vi "UTILITY Build Save Array.vi"(8 "Error In":errorcluster, 10 "New Header Save Array":T1[](array[typedef]), 11 "Full Data Array Out":string[][](array[string])) -> (0 "Error Out":errorcluster, 3 "Selected Data Array Out":string[][](array[string]))   [LabVIEW 2016]
uses:
  Washer DOE/Type Definitions/DOE Data Save Modifier.ctl
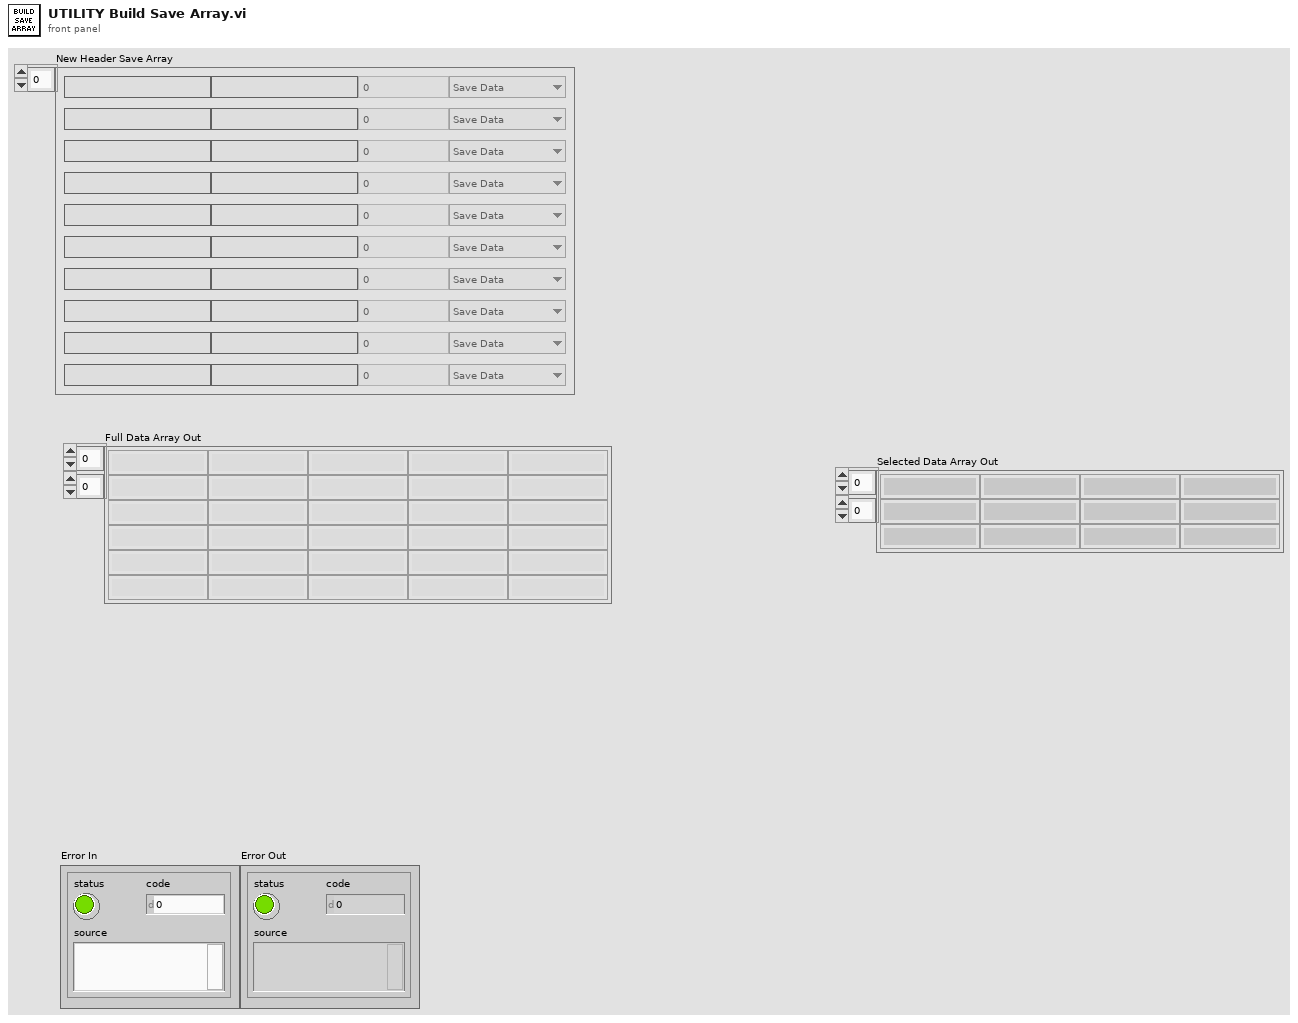
[diagram p1: front panel]
types:
  T1 = typedef "DOE Data Save Modifier.ctl" = cluster{"Name":string, "Title":string, "Save Status":enum16{"Save Data", "Don't Save Data"}, "Group":u8, "Field":u8}
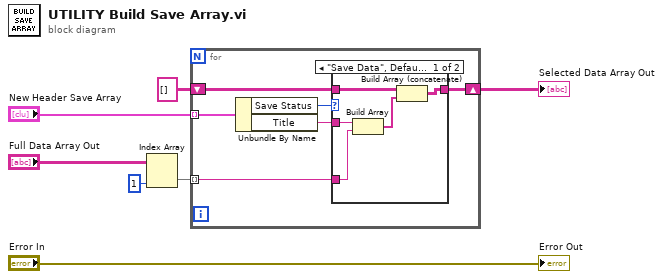
[diagram p0: block diagram]
diagram:
  n1 = Index Array(array="Full Data Array Out", index (col)=1 ("index (row)")) -> (element=w3:string[])  [unwired: 1 in]
  n2 = for {
    tunnel: "New Header Save Array" -> [w13] mode=indexing
    shift-right: [w10] -> w2
    shift-left: string[][] [] -> [w11]
    tunnel: w3 -> [w8] mode=indexing
    n3 = Unbundle By Name(w13) -> ("Save Status"=w12:enum16{"Save Data", "Don't Save Data"}, "Title"=w9:string)
    n4 = case shown="\"Save Data\", Default" w12 {
      tunnel: w11 -> [w18 w19]
      tunnel: [w17 w19] -> w10
      tunnel: w9 -> [w16 _]
      tunnel: w8 -> [w15 _]
      frame "Save Data", Default {
        n5 = Build Array(w16, w15) -> (w14:string[])
        n6 = Build Array (concatenate)(w18, w14) -> (w17:string[][])
      }
      frame "Don't Save Data" {
      }
    }
  }
  "Selected Data Array Out" <- w2
  "Error Out" <- "Error In"
